vi "Get Configuration Session.vi"(8 "error in (no error)":errorcluster, 11 "Item Ref in":T1 format="%.0x") -> (0 "error out":errorcluster, 2 "Configuration Session":refnum<class "Configuration Session.lvclass">, 3 "Item Ref out":T1 format="%.0x")   [LabVIEW 2017, in "DSF System Explorer.lvlib"]
uses:
  DSF System Explorer.lvlib
  <vilib>/NI Veristand/Custom Device API/Custom Device Item Ref.ctl
  DSF Core.lvlibp/Classes/Configuration/Configuration Session.lvclass
  <vilib>/NI Veristand/Custom Device API/Custom Device API.lvlib
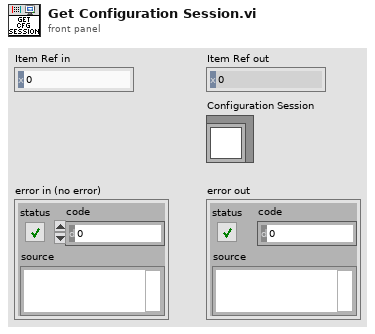
[diagram p1: front panel]
types:
  T1 = typedef "Custom Device API.lvlib/Custom Device Item Ref.ctl" = u64
  T2 = typedef "DSF System Explorer.lvlib/shared data.ctl" = cluster{"Configuration Session":refnum<class "Configuration Session.lvclass">}
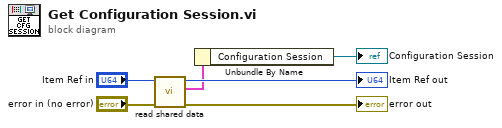
[diagram p0: block diagram]
diagram:
  n1 = call "read shared data.vi"("error in (no error)"="error in (no error)", "Item Ref in"="Item Ref in") -> ("error out"=→"error out":errorcluster, "shared data"=w1:T2, "Item Ref out"=→"Item Ref out":T1)  [unwired: 7 in]
  n2 = Unbundle By Name(w1) -> ("Configuration Session"=→"Configuration Session":refnum<class "Configuration Session.lvclass">)
